vi "start.vi"(8 "error in (no error)":errorcluster, 11 "FPGA_AK101022Resonance in":refnum<class "FPGAWrapperAK101022Resonance.lvclass">) -> (0 "error out":errorcluster, 3 "FPGA_AK101022Resonance out":refnum<class "FPGAWrapperAK101022Resonance.lvclass">)   [LabVIEW 2010, in "FPGAWrapperAK101022Resonance.lvclass"]
uses:
  FPGAWrapperAK101022Resonance.lvclass
  class_data.vi
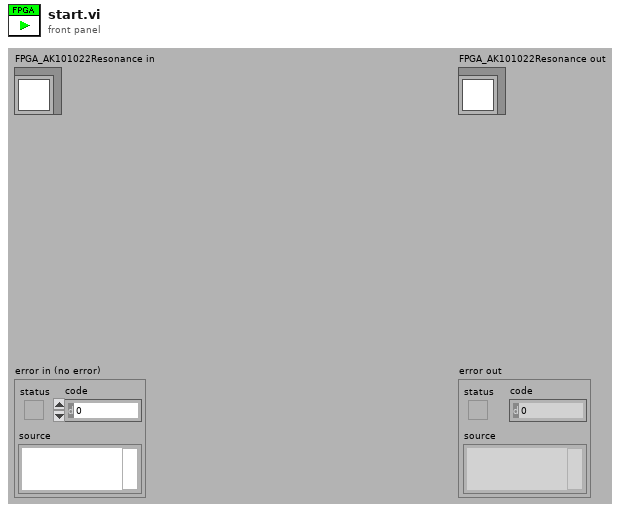
[diagram p1: front panel]
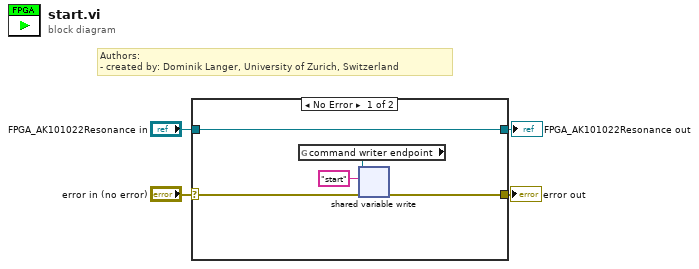
[diagram p0: block diagram]
diagram:
  # "Authors: \n- created by: Dominik Langer, University of Zurich, Switzerland"
  n1 = case shown="No Error" "error in (no error)" {
    selector: "error in (no error)" -> [w6 w10]
    tunnel: "FPGA_AK101022Resonance in" -> [w8 w11]
    tunnel: [w9 w10] -> w2
    tunnel: [w8 w11] -> w1
    frame No Error {
      n2 = global read "class_data.vi" "command writer endpoint"() -> (w7:refnum<k21>)
      n3 = shared-variable-write(w7, w6, "start" ("data in")) -> (w9:errorcluster)  [unwired: 1 in, 2 out]
    }
    frame Error {
    }
  }
  "error out" <- w2
  "FPGA_AK101022Resonance out" <- w1
